vi "InitBaseMission.vi"(11 "Boat Location":refnum<notifier>) -> (3 "Mission Array":refnum<class "Idle.lvclass">[](array[class]))   [LabVIEW 2013]
doc: "This VI initializes a base mission (Idle at point) at the indicated boat position. Unimplemented possibilities:\n1) Choose the desired idle point at the beeginning\n2) Idle where the boat starts\nThis VI was mostly created to clean up Forebrain Main.\n\nEric Schneider, August 2014"
uses:
  Data/TypeDefs/UTM Location.ctl
  Classes/Missions/Idle/Idle.lvclass
  Data/TypeDefs/MissionTypeControl.ctl
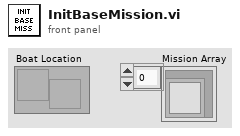
[diagram p1: front panel]
types:
  T1 = typedef "MissionTypeControl.ctl" = enum16{"Idle at Point", "Drive to Waypoint", "Round Buoy to Port", "Round Buoy to Starboard", "Pass Between Buoys", "Station Keeping"}
  T2 = typedef "UTM Location.ctl" = cluster{"UTM Zone":dbl, "Hemisphere":enum16{"North", "South"}, "East":dbl, "North":dbl}
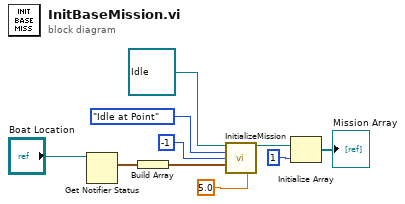
[diagram p0: block diagram]
diagram:
  n1 = Get Notifier Status(notifier="Boat Location") -> (current notification=w6:T2)  [unwired: 1 in, 4 out]
  n2 = Build Array(w6) -> (w7:T2[])
  n3 = call-dynamic "InitializeMission.vi"("GenericMission in"=refnum<class "Idle.lvclass"> refnum ("Idle.lvclass"), "Mission Type"=MissionTypeControl."Idle at Point", "ID#"=i16 -1, "Points of Interest"=w7, "Tolerance (m)"=5.0) -> ("GenericMission out"=w4:refnum<class "Idle.lvclass">)  [unwired: 9 in, 1 out]
  n4 = Initialize Array(w4, 1 ("dimension size")) -> (→"Mission Array":refnum<class "Idle.lvclass">[])
